vi "use of local variables in loops.vi"() -> ()   [LabVIEW 2012]
panel:
  out "number (0 to 1) 2":dbl
  out "number (0 to 1)":dbl
  in  "stop":bool
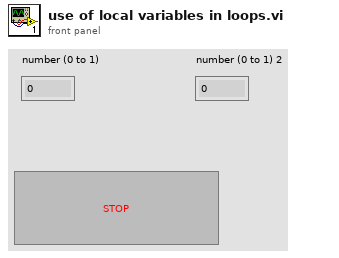
[diagram p1: front panel]
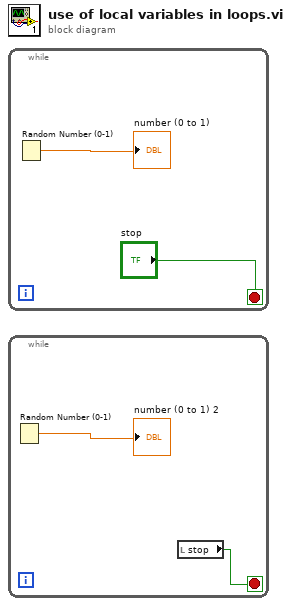
[diagram p0: block diagram]
diagram:
  n1 = while {
    stop <- "stop" stop-if-true
    n2 = Random Number (0-1)() -> (number: 0 to 1=→"number (0 to 1)":dbl)
  }
  n3 = while {
    stop <- w3 stop-if-true
    n4 = Random Number (0-1)() -> (number: 0 to 1=→"number (0 to 1) 2":dbl)
    n5 = local read "stop"() -> (w3:bool)
  }
